vi "Exercise 4.1 - Manual Analysis.vi"() -> ()   [LabVIEW 2012]
panel:
  out "Frequency":dbl
  out "Amplitude":dbl
  in  "Frequency In":dbl(knob)=14.491987418089225 scale=0.0..100.0
  out "Waveform Graph":dynamicdata(graph)
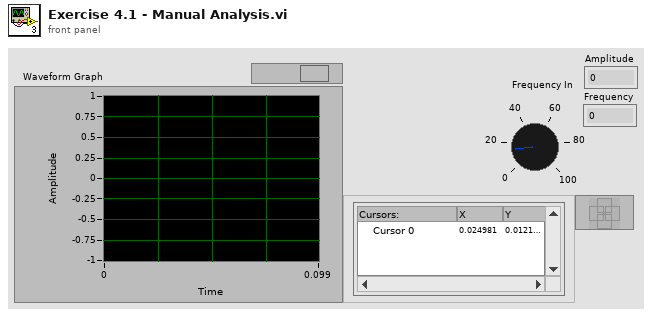
[diagram p1: front panel]
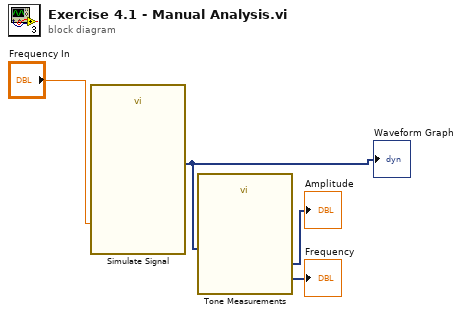
[diagram p0: block diagram]
diagram:
  n1 = call "Simulate Signal"("Frequency"="Frequency In") -> ("Sine"=w1:dynamicdata)  [unwired: 13 in, 1 out]
  "Waveform Graph" <- w1
  n2 = call "Tone Measurements"("Signals"=w1) -> ("Frequency"=→"Frequency":dynamicdata, "Amplitude"=→"Amplitude":dynamicdata)  [unwired: 8 in, 1 out]
